vi "CRYGet Data by Name.vi"(6 "Type":enum16{"Curves", "Values", "Results", "WFM"}(ring), 8 "sOption":string, 9 "AutoProtected Index":i32[](array[numeric]), 10 "Data Names":string[](array[string]), 11 "pVIGraph In":refnum<vi>) -> (0 "Item Symbols":i32[](array[numeric]), 1 "Value Rows":i32[](array[numeric]), 2 "Curve Rows":i32[](array[numeric]), 3 "Replot?":bool, 4 "Result Rows":i32[](array[numeric]), 5 "pGraph VI Out":refnum<vi>, 7 "bSameRemainReplot":bool)   [LabVIEW 2013]
uses:
  CRYCurveLibrary/Global/CRYCurve Library Global.vi
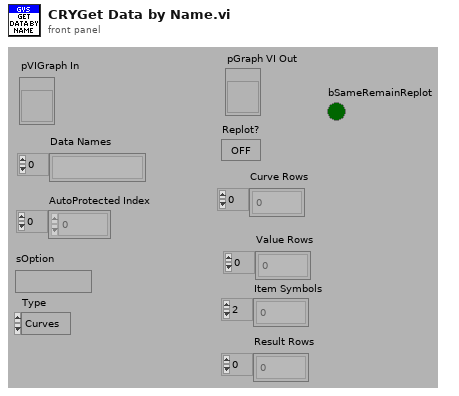
[diagram p1: front panel]
types:
  T1 = cluster{"Curve Index":i32[], "Value Index":i32[], "Result Index":i32[], "WFM Index":i32[], "Curve Names":string[], "Value Names":string[], "Result Names":string[], "WFM Names":string[]}
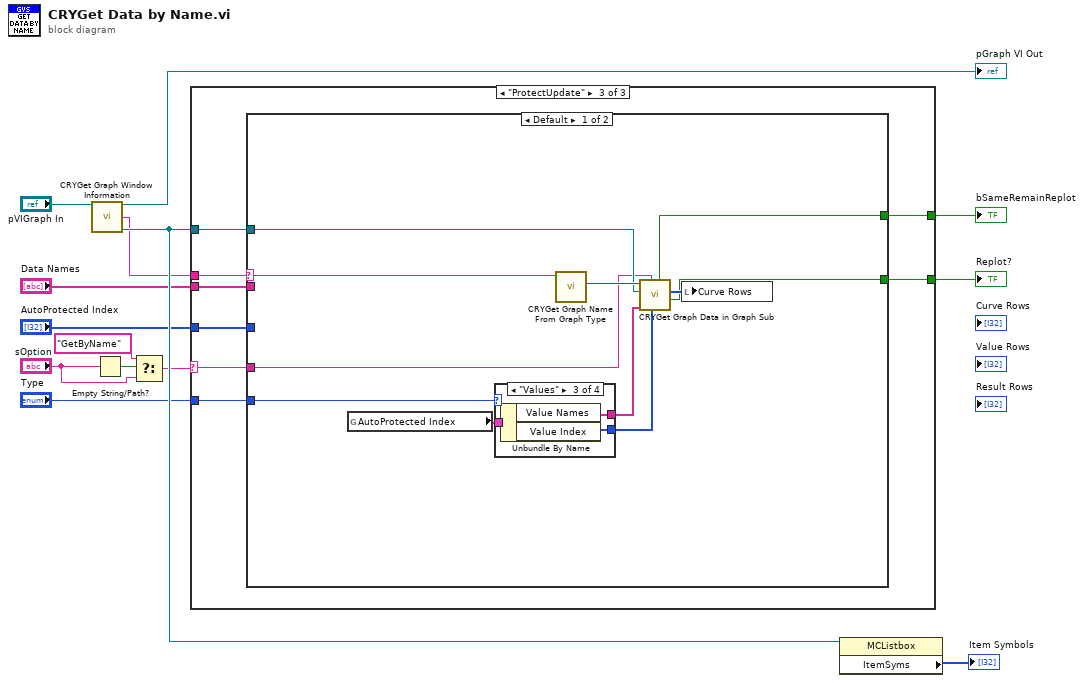
[diagram p0: block diagram]
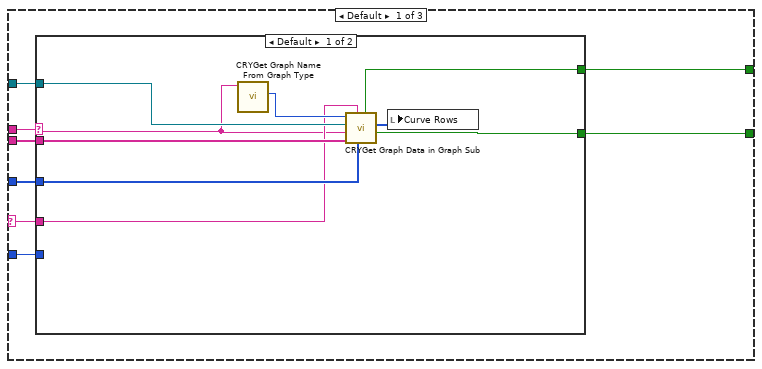
[diagram p2: hidden frame]
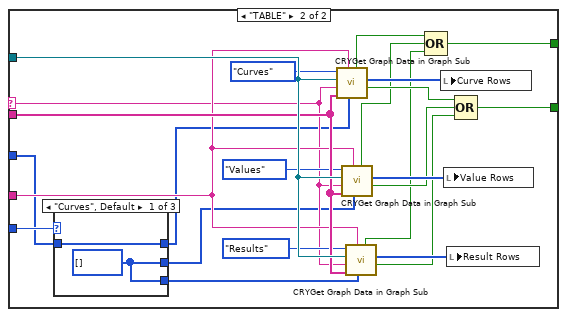
[diagram p3: hidden frame]
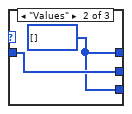
[diagram p4: hidden frame]
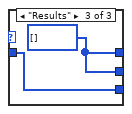
[diagram p5: hidden frame]
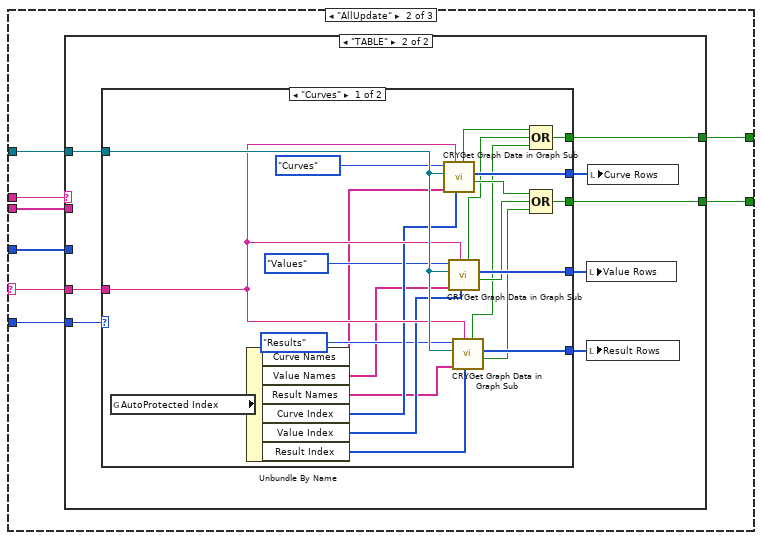
[diagram p6: hidden frame]
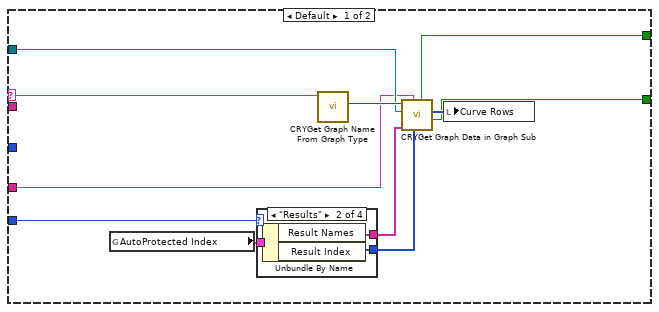
[diagram p7: hidden frame]
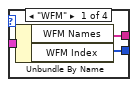
[diagram p8: hidden frame]
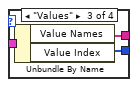
[diagram p9: hidden frame]
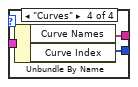
[diagram p10: hidden frame]
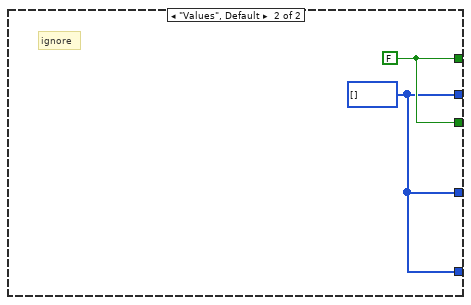
[diagram p11: hidden frame]
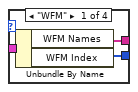
[diagram p12: hidden frame]
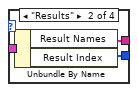
[diagram p13: hidden frame]
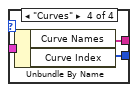
[diagram p14: hidden frame]
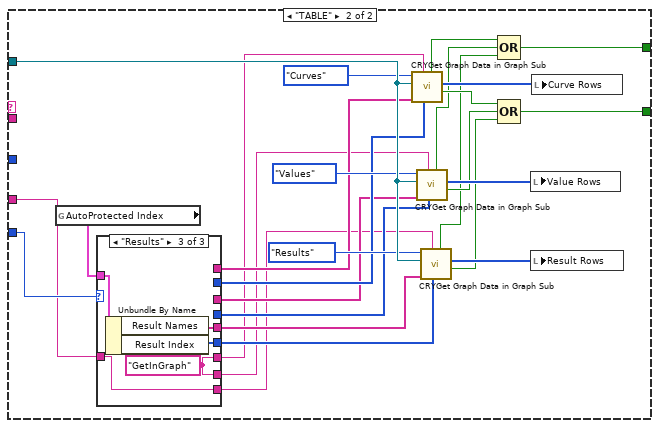
[diagram p15: hidden frame]
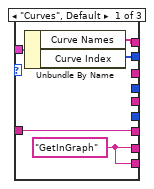
[diagram p16: hidden frame]
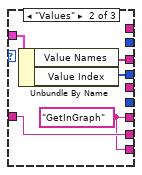
[diagram p17: hidden frame]
diagram:
  n1 = call "CRYGet Graph Window Information.vi"("pGraph VI In"="pVIGraph In") -> ("pGraph VI Out"=→"pGraph VI Out":refnum<vi>, "Graph Type Out"=w9:string, "Legend Ref Out"=w11:refnum<vi>)  [unwired: 2 in, 10 out]
  n2 = Empty String/Path?(string/path="sOption") -> (empty?=w6:bool)
  n3 = Select(t="GetByName" ("sAction"), s=w6, f="sOption") -> (s? t:f=w3:string)
  n4 = case shown="\"ProtectUpdate\"" w3 {
    selector: w3 -> [w17 w62 w126]
    tunnel: w11 -> [w22 w68 w132]
    tunnel: "Data Names" -> [w21 w67 w131]
    tunnel: w9 -> [w20 w66 w130]
    tunnel: [w19 w65 w129] -> w8
    tunnel: "AutoProtected Index" -> [w18 w64 w128]
    tunnel: "Type" -> [w15 w63 w127]
    tunnel: [w16 w61 w125] -> w2
    frame Default {
      n5 = case shown="Default" w20 {
        selector: w20 -> [w23 w37]
        tunnel: w22 -> [w30 w53]
        tunnel: w21 -> [w29 w52]
        tunnel: [w27 w54] -> w19
        tunnel: w18 -> [w26 w35]
        tunnel: w17 -> [w25 w48]
        tunnel: [w24 w38] -> w16
        tunnel: w15 -> [_ w36]
        frame Default {
          n6 = call "CRYGet Graph Name From Graph Type.vi"("Graph Type"=w23) -> ("Type"=w31:enum16{"Curves", "Values", "Results", "WFM"})  [unwired: 9 in, 1 out]
          n7 = call "CRYGet Graph Data in Graph Sub.vi"("Index"=w26, "sOption"=w25, "Data Names"=w29, "sGraphType"=w23, "Legend Refnum"=w30, "Type In"=w31) -> ("bResult"=w27:bool, "Rows"=w28:i32[], "bSameRemainReplot"=w24:bool)  [unwired: 1 in, 2 out]
          n8 = local write "Curve Rows"(w28) -> ()
        }
        frame "TABLE" {
          n9 = case shown="\"Curves\", Default" w36 {
            tunnel: w35 -> [w56 w58 w59]
            tunnel: [w56 w57 w60] -> w34
            tunnel: [w55 w58 w60] -> w33
            tunnel: [w55 w57 w59] -> w32
            frame "Curves", Default {
              w55 = i32[] [] ("AutoProtected Index")
            }
            frame "Values" {
              w57 = i32[] [] ("AutoProtected Index")
            }
            frame "Results" {
              w60 = i32[] [] ("AutoProtected Index")
            }
          }
          n10 = call "CRYGet Graph Data in Graph Sub.vi"("Index"=w34, "sOption"=w48, "Data Names"=w52, "sGraphType"=w37, "Legend Refnum"=w53, "Type In"=enum16{"Curves", "Values", "Results", "WFM"}."Curves") -> ("bResult"=w45:bool, "Rows"=w51:i32[], "bSameRemainReplot"=w41:bool)  [unwired: 1 in, 2 out]
          n11 = call "CRYGet Graph Data in Graph Sub.vi"("Index"=w33, "sOption"=w48, "Data Names"=w52, "sGraphType"=w37, "Legend Refnum"=w53, "Type In"=enum16{"Curves", "Values", "Results", "WFM"}."Values") -> ("bResult"=w44:bool, "Rows"=w50:i32[], "bSameRemainReplot"=w40:bool)  [unwired: 1 in, 2 out]
          n12 = call "CRYGet Graph Data in Graph Sub.vi"("Index"=w32, "sOption"=w48, "Data Names"=w52, "sGraphType"=w37, "Legend Refnum"=w53, "Type In"=enum16{"Curves", "Values", "Results", "WFM"}."Results") -> ("bResult"=w42:bool, "Rows"=w49:i32[], "bSameRemainReplot"=w39:bool)  [unwired: 1 in, 2 out]
          n13 = Compound Arithmetic op=OR(w41, w40, w39) -> (w38:bool)
          n14 = local write "Curve Rows"(w51) -> ()
          n15 = local write "Value Rows"(w50) -> ()
          n16 = local write "Result Rows"(w49) -> ()
          n17 = Compound Arithmetic op=OR(w45, w44, w42) -> (w54:bool)
        }
      }
    }
    frame "AllUpdate" {
      n18 = case shown="\"TABLE\"" w66 {
        selector: w66 -> [w74 _]
        tunnel: w68 -> [w78 w98]
        tunnel: w67 -> [_ _]
        tunnel: [w76 w99] -> w65
        tunnel: w64 -> [_ _]
        tunnel: w62 -> [w75 w94]
        tunnel: w63 -> [w72 w92]
        tunnel: [w69 w93] -> w61
        frame Default {
          n19 = global read "CRYCurve Library Global.vi" "AutoProtected Index"() -> (w73:T1)
          n20 = case shown="\"Results\"" w72 {
            tunnel: w73 -> [w82 w85 w88 w91]
            tunnel: [w81 w84 w87 w90] -> w71
            tunnel: [w80 w83 w86 w89] -> w70
            frame "WFM" {
              n21 = Unbundle By Name(w82) -> ("WFM Names"=w80:string[], "WFM Index"=w81:i32[])
            }
            frame "Results" {
              n22 = Unbundle By Name(w85) -> ("Result Names"=w83:string[], "Result Index"=w84:i32[])
            }
            frame "Values" {
              n23 = Unbundle By Name(w88) -> ("Value Names"=w86:string[], "Value Index"=w87:i32[])
            }
            frame "Curves" {
              n24 = Unbundle By Name(w91) -> ("Curve Names"=w89:string[], "Curve Index"=w90:i32[])
            }
          }
          n25 = call "CRYGet Graph Name From Graph Type.vi"("Graph Type"=w74) -> ("Type"=w79:enum16{"Curves", "Values", "Results", "WFM"})  [unwired: 9 in, 1 out]
          n26 = call "CRYGet Graph Data in Graph Sub.vi"("Index"=w71, "sOption"=w75, "Data Names"=w70, "Legend Refnum"=w78, "Type In"=w79) -> ("bResult"=w76:bool, "Rows"=w77:i32[], "bSameRemainReplot"=w69:bool)  [unwired: 2 in, 2 out]
          n27 = local write "Curve Rows"(w77) -> ()
        }
        frame "TABLE" {
          n28 = case shown="\"Curves\"" w92 {
            tunnel: [w122 w124] -> w99
            tunnel: w98 -> [w121 _]
            tunnel: [w120 w123] -> w97
            tunnel: [w119 w123] -> w96
            tunnel: [w118 w123] -> w95
            tunnel: w94 -> [w117 _]
            tunnel: [w116 w124] -> w93
            frame "Curves" {
              n29 = global read "CRYCurve Library Global.vi" "AutoProtected Index"() -> (w112:T1)
              n30 = Unbundle By Name(w112) -> ("Curve Names"=w103:string[], "Value Names"=w104:string[], "Result Names"=w105:string[], "Curve Index"=w111:i32[], "Value Index"=w110:i32[], "Result Index"=w109:i32[])
              n31 = call "CRYGet Graph Data in Graph Sub.vi"("Index"=w111, "sOption"=w117, "Data Names"=w103, "Legend Refnum"=w121, "Type In"=enum16{"Curves", "Values", "Results", "WFM"}."Curves") -> ("bResult"=w115:bool, "Rows"=w120:i32[], "bSameRemainReplot"=w102:bool)  [unwired: 2 in, 2 out]
              n32 = call "CRYGet Graph Data in Graph Sub.vi"("Index"=w110, "sOption"=w117, "Data Names"=w104, "Legend Refnum"=w121, "Type In"=enum16{"Curves", "Values", "Results", "WFM"}."Values") -> ("bResult"=w114:bool, "Rows"=w119:i32[], "bSameRemainReplot"=w101:bool)  [unwired: 2 in, 2 out]
              n33 = call "CRYGet Graph Data in Graph Sub.vi"("Index"=w109, "sOption"=w117, "Data Names"=w105, "Legend Refnum"=w121, "Type In"=enum16{"Curves", "Values", "Results", "WFM"}."Results") -> ("bResult"=w113:bool, "Rows"=w118:i32[], "bSameRemainReplot"=w100:bool)  [unwired: 2 in, 2 out]
              n34 = Compound Arithmetic op=OR(w102, w101, w100) -> (w116:bool)
              n35 = Compound Arithmetic op=OR(w115, w114, w113) -> (w122:bool)
            }
            frame "Values", Default {
              w123 = i32[] [] ("Rows")
              w124 = FALSE
              # "ignore"
            }
          }
          n36 = local write "Value Rows"(w96) -> ()
          n37 = local write "Result Rows"(w95) -> ()
          n38 = local write "Curve Rows"(w97) -> ()
        }
      }
    }
    frame "ProtectUpdate" {
      n39 = case shown="Default" w130 {
        selector: w130 -> [w138 _]
        tunnel: w132 -> [w142 w181]
        tunnel: w131 -> [_ _]
        tunnel: [w140 w182] -> w129
        tunnel: w128 -> [_ _]
        tunnel: w126 -> [w139 w159]
        tunnel: w127 -> [w136 w167]
        tunnel: [w133 w177] -> w125
        frame Default {
          n40 = global read "CRYCurve Library Global.vi" "AutoProtected Index"() -> (w137:T1)
          n41 = case shown="\"Values\"" w136 {
            tunnel: w137 -> [w146 w149 w152 w155]
            tunnel: [w145 w148 w151 w154] -> w135
            tunnel: [w144 w147 w150 w153] -> w134
            frame "WFM" {
              n42 = Unbundle By Name(w146) -> ("WFM Names"=w144:string[], "WFM Index"=w145:i32[])
            }
            frame "Results" {
              n43 = Unbundle By Name(w149) -> ("Result Names"=w147:string[], "Result Index"=w148:i32[])
            }
            frame "Values" {
              n44 = Unbundle By Name(w152) -> ("Value Names"=w150:string[], "Value Index"=w151:i32[])
            }
            frame "Curves" {
              n45 = Unbundle By Name(w155) -> ("Curve Names"=w153:string[], "Curve Index"=w154:i32[])
            }
          }
          n46 = call "CRYGet Graph Name From Graph Type.vi"("Graph Type"=w138) -> ("Type"=w143:enum16{"Curves", "Values", "Results", "WFM"})  [unwired: 9 in, 1 out]
          n47 = call "CRYGet Graph Data in Graph Sub.vi"("Index"=w135, "sOption"=w139, "Data Names"=w134, "Legend Refnum"=w142, "Type In"=w143) -> ("bResult"=w140:bool, "Rows"=w141:i32[], "bSameRemainReplot"=w133:bool)  [unwired: 2 in, 2 out]
          n48 = local write "Curve Rows"(w141) -> ()
        }
        frame "TABLE" {
          n49 = global read "CRYCurve Library Global.vi" "AutoProtected Index"() -> (w166:T1)
          n50 = case shown="\"Results\"" w167 {
            tunnel: w166 -> [w187 w192 w197]
            tunnel: [w186 _ _] -> w165
            tunnel: [w185 _ _] -> w164
            tunnel: [w183 w189 w194] -> w157
            tunnel: [_ w191 _] -> w163
            tunnel: [_ w190 _] -> w160
            tunnel: [_ _ w196] -> w162
            tunnel: [_ _ w195] -> w161
            tunnel: w159 -> [w184 w189 w193]
            tunnel: [w184 w188 w194] -> w158
            tunnel: [w183 w188 w193] -> w156
            frame "Curves", Default {
              w183 = "GetInGraph"
              n51 = Unbundle By Name(w187) -> ("Curve Names"=w186:string[], "Curve Index"=w185:i32[])
            }
            frame "Values" {
              w188 = "GetInGraph"
              n52 = Unbundle By Name(w192) -> ("Value Names"=w191:string[], "Value Index"=w190:i32[])
            }
            frame "Results" {
              w194 = "GetInGraph"
              n53 = Unbundle By Name(w197) -> ("Result Names"=w196:string[], "Result Index"=w195:i32[])
            }
          }
          n54 = call "CRYGet Graph Data in Graph Sub.vi"("Index"=w164, "sOption"=w158, "Data Names"=w165, "Legend Refnum"=w181, "Type In"=enum16{"Curves", "Values", "Results", "WFM"}."Curves") -> ("bResult"=w176:bool, "Rows"=w180:i32[], "bSameRemainReplot"=w170:bool)  [unwired: 2 in, 2 out]
          n55 = call "CRYGet Graph Data in Graph Sub.vi"("Index"=w160, "sOption"=w157, "Data Names"=w163, "Legend Refnum"=w181, "Type In"=enum16{"Curves", "Values", "Results", "WFM"}."Values") -> ("bResult"=w175:bool, "Rows"=w179:i32[], "bSameRemainReplot"=w169:bool)  [unwired: 2 in, 2 out]
          n56 = call "CRYGet Graph Data in Graph Sub.vi"("Index"=w161, "sOption"=w156, "Data Names"=w162, "Legend Refnum"=w181, "Type In"=enum16{"Curves", "Values", "Results", "WFM"}."Results") -> ("bResult"=w174:bool, "Rows"=w178:i32[], "bSameRemainReplot"=w168:bool)  [unwired: 2 in, 2 out]
          n57 = Compound Arithmetic op=OR(w170, w169, w168) -> (w177:bool)
          n58 = Compound Arithmetic op=OR(w176, w175, w174) -> (w182:bool)
          n59 = local write "Value Rows"(w179) -> ()
          n60 = local write "Result Rows"(w178) -> ()
          n61 = local write "Curve Rows"(w180) -> ()
        }
      }
    }
  }
  "Replot?" <- w8
  "bSameRemainReplot" <- w2
  n62 = property class="MCListbox"(reference=w11) -> ("ItemSyms"=→"Item Symbols":i32[])  [unwired: 1 in, 2 out]
